vi "NOx test MAX FPGA.vi"() -> ()   [LabVIEW 2011]
uses:
  <vilib>/rvi/eio/common/nirviEmuTemplateMethod_errors.vi
  <vilib>/eio/EIONode/EIONode.xnode
  <vilib>/LabVIEW Targets/FPGA/RIO/nicrio_985x_controls.llb/CAN_IO_Frame Cluster.ctl
  <vilib>/LabVIEW Targets/FPGA/RIO/nicrio_985x_controls.llb/CAN_IO_Frame Type.ctl
panel:
  out "NOxSensorData 2":T1={"NOx (bits)"=0, "O2 (bits)"=0, "Sensor Supply Status"=3, "Sensor Temperature Status"=12, "NOx Signal Status"=48, "O2 Signal Status"=192, "Heater Mode Status"=96, "Heater Circuit Status"=31, "NOx Circuit Status"=31, "O2 Circuit Status"=31, "NOx Sensor Module Present"=FALSE} {"Heater Mode Status" items=["AUTO MODE"=0, "HEATUP SLOPE 3 OR 4"=32, "HEATUP SLOPE 1 OR 2"=64, "HEATER OFF / PREHEAT"=96]; "O2 Circuit Status" items=["OPEN WIRE"=3, "SHORT CIRCUIT"=5, "NO ERROR"=31]; "NOx Circuit Status" items=["OPEN WIRE"=3, "SHORT CIRCUIT"=5, "NO ERROR"=31]; "Heater Circuit Status" items=["OPEN WIRE"=3, "SHORT CIRCUIT"=5, "NO ERROR"=31]; "Sensor Temperature Status" items=["NOT AT TEMPERATURE"=0, "AT TEMPERATURE"=4, "ERROR"=8, "NOT AVAILABLE"=12]; "O2 Signal Status" items=["NOT VALID"=0, "VALID"=64, "ERROR"=128, "NOT AVAILABLE"=192]; "NOx Signal Status" items=["NOT VALID"=0, "VALID"=16, "ERROR"=32, "NOT AVAILABLE"=48]; "Sensor Supply Status" items=["NOT IN RANGE", "SUPPLY IN RANGE", "ERROR", "NOT AVAILABLE"]}
  out "NOxSensorData 1":T1={"NOx (bits)"=0, "O2 (bits)"=0, "Sensor Supply Status"=3, "Sensor Temperature Status"=12, "NOx Signal Status"=48, "O2 Signal Status"=192, "Heater Mode Status"=96, "Heater Circuit Status"=31, "NOx Circuit Status"=31, "O2 Circuit Status"=31, "NOx Sensor Module Present"=FALSE} {"Heater Mode Status" items=["AUTO MODE"=0, "HEATUP SLOPE 3 OR 4"=32, "HEATUP SLOPE 1 OR 2"=64, "HEATER OFF / PREHEAT"=96]; "O2 Circuit Status" items=["OPEN WIRE"=3, "SHORT CIRCUIT"=5, "NO ERROR"=31]; "NOx Circuit Status" items=["OPEN WIRE"=3, "SHORT CIRCUIT"=5, "NO ERROR"=31]; "Heater Circuit Status" items=["OPEN WIRE"=3, "SHORT CIRCUIT"=5, "NO ERROR"=31]; "Sensor Temperature Status" items=["NOT AT TEMPERATURE"=0, "AT TEMPERATURE"=4, "ERROR"=8, "NOT AVAILABLE"=12]; "O2 Signal Status" items=["NOT VALID"=0, "VALID"=64, "ERROR"=128, "NOT AVAILABLE"=192]; "NOx Signal Status" items=["NOT VALID"=0, "VALID"=16, "ERROR"=32, "NOT AVAILABLE"=48]; "Sensor Supply Status" items=["NOT IN RANGE", "SUPPLY IN RANGE", "ERROR", "NOT AVAILABLE"]}
  in  "Sensor2Enable":bool=TRUE
  in  "RxID 1":u32=418385746 format="%08x"
  in  "TxID":u32=419356416 format="%08x"
  in  "Sensor1Enable":bool=TRUE
  in  "RxID 2":u32=418385489 format="%08x"
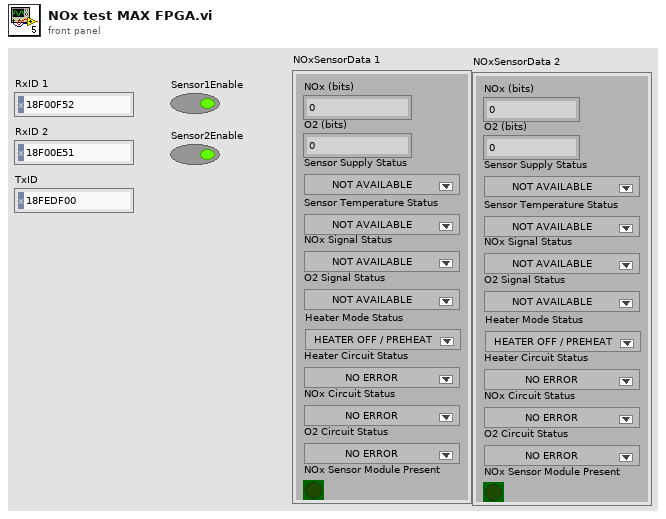
[diagram p1: front panel]
types:
  T1 = cluster{"NOx (bits)":u16, "O2 (bits)":u16, "Sensor Supply Status":u8, "Sensor Temperature Status":u8, "NOx Signal Status":u8, "O2 Signal Status":u8, "Heater Mode Status":u8, "Heater Circuit Status":u8, "NOx Circuit Status":u8, "O2 Circuit Status":u8, "NOx Sensor Module Present":bool}
  T2 = typedef "CAN_IO_Frame Cluster.ctl" = cluster{"timestamp high":u32, "timestamp low":u32, "identifier":u32, "type":T3, "info A":u8, "info B":u8, "data length":u8, "data":u8[]}
  T3 = typedef "CAN_IO_Frame Type.ctl" = enum8{"Data Frame", "Remote Frame", "(reserved)", "(reserved) ", "(reserved)  ", "(reserved)   ", "Bus Error", "Transceiver Fault"}
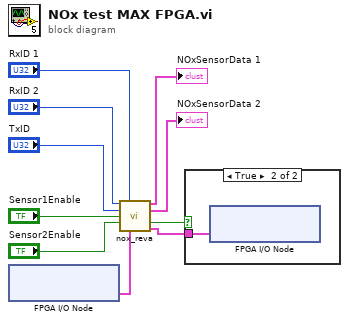
[diagram p0: block diagram]
diagram:
  n1 = xnode "FPGA I/O Node"() -> ("Mod5/CAN0"=w5:T2)  [unwired: 1 in, 1 out]
  n2 = call <vilib>:"nox_reva.vi"("RxID 2"="RxID 2", "RxID 1"="RxID 1", "TxID"="TxID", "Sensor1Enable"="Sensor1Enable", "Sensor2Enable"="Sensor2Enable", "CAN Data In"=w5) -> ("NOxSensorData 1"=→"NOxSensorData 1":T1, "NOxSensorData 2"=→"NOxSensorData 2":T1, "Update CAN Out"=w3:bool, "CAN Data Out"=w4:T2)  [unwired: 5 in, 1 out]
  n3 = case shown="True" w3 {
    tunnel: w4 -> [_ w11]
    frame False {
    }
    frame True {
      n4 = xnode "FPGA I/O Node"("Mod5/CAN0"=w11) -> ()  [unwired: 1 in, 1 out]
    }
  }
